vi "ParseXMLComment4Params.vi"(8 "error in":errorcluster, 11 "XML Comment":string) -> (0 "error out":errorcluster, 3 "ARINC Parameter":T1)   [LabVIEW 2011, in "AIT 429 Custom Device.lvlib"]
uses:
  AIT 429 Custom Device.lvlib
  Controls/ARINCParam.ctl
  <vilib>/xml/Close Reference(Node).vi
  Program Files (x86)/National Instruments/LabVIEW 2011/resource/objmgr/DOMUserDefRef.rc
  <vilib>/xml/NI_XML.lvlib
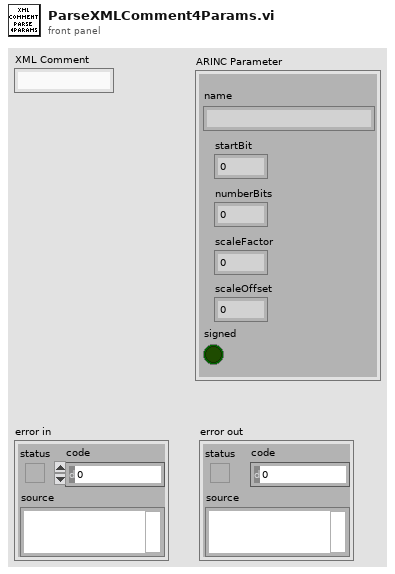
[diagram p1: front panel]
types:
  T1 = typedef "AIT 429 Custom Device.lvlib/ARINCParam.ctl" = cluster{"name":string, "startBit":i32, "numberBits":i32, "scaleFactor":dbl, "scaleOffset":dbl, "signed":bool}
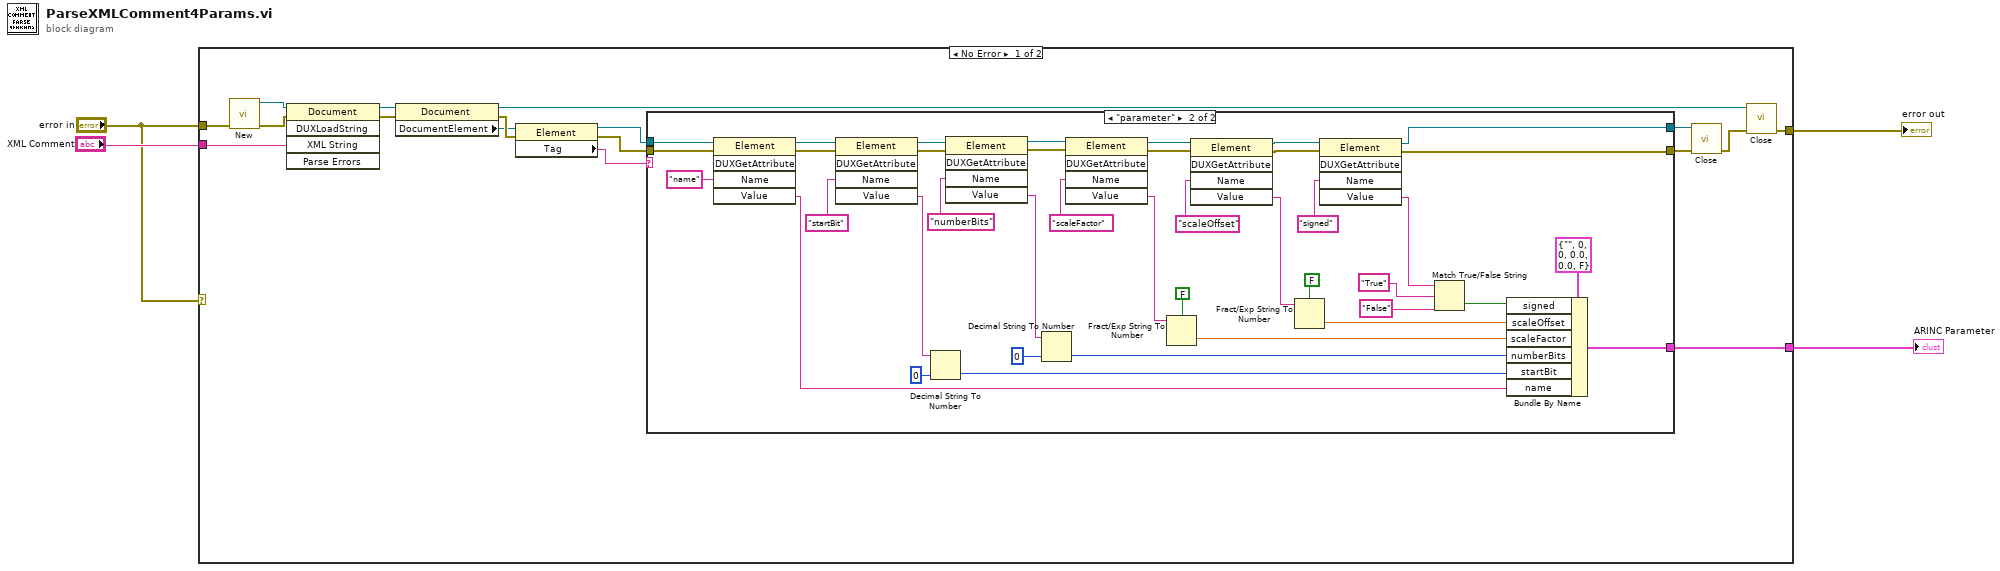
[diagram p0: block diagram]
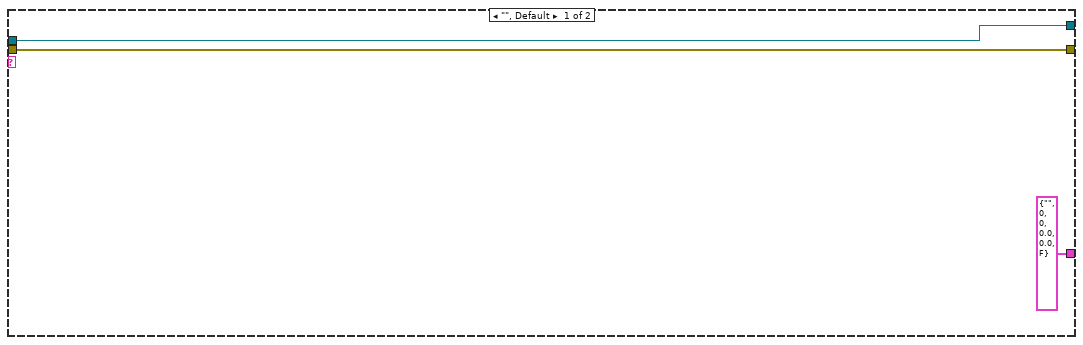
[diagram p2: hidden frame]
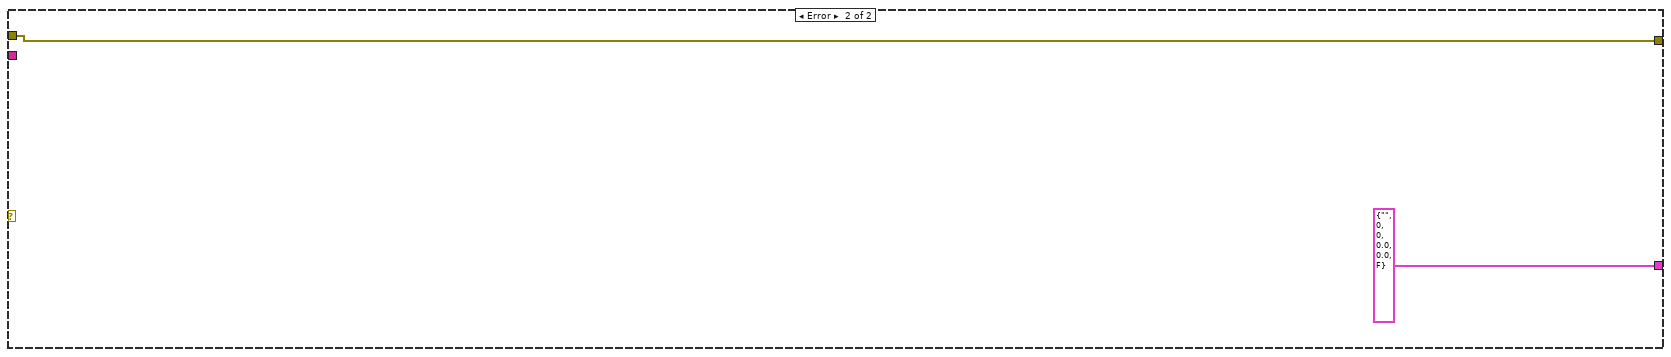
[diagram p3: hidden frame]
diagram:
  n1 = case shown="No Error" "error in" {
    tunnel: [w16 w65] -> w4
    tunnel: "XML Comment" -> [w9 _]
    tunnel: "error in" -> [w8 w65]
    tunnel: [w5 T1 {"name"="", "startBit"=0, "numberBits"=0, "scaleFactor"=0.0, "scaleOffset"=0.0, "signed"=FALSE} ("ARINC Parameter")] -> w2
    frame No Error {
      n2 = call <vilib>:"New.vi"("error in (no error)"=w8) -> ("error out"=w10:errorcluster, "DOM document out"=w7:refnum<k20>)  [unwired: 7 in]
      n3 = invoke class="Document" method="DUXLoadString"(reference=w7, error in=w10, "XML String"=w9) -> (reference out=w6:refnum<k20>, error out=w11:errorcluster)  [unwired: 2 in, 3 out]
      n4 = property on="Property Node" class="Document"(reference=w6, error in=w11) -> (reference out=w12:refnum<k20>, error out=w19:errorcluster, "DocumentElement"=w17:refnum<k20>)
      n5 = property class="Element"(reference=w17, error in=w19) -> (reference out=w18:refnum<k20>, error out=w20:errorcluster, "Tag"=w21:string)
      n6 = case shown="\"parameter\"" w21 {
        tunnel: [w23 w31] -> w14
        tunnel: [w24 w32] -> w15
        tunnel: w18 -> [w23 w62]
        tunnel: w20 -> [w24 w61]
        tunnel: [T1 {"name"="", "startBit"=0, "numberBits"=0, "scaleFactor"=0.0, "scaleOffset"=0.0, "signed"=FALSE} ("ARINC Parameter") w27] -> w5
        frame "", Default {
        }
        frame "parameter" {
          n7 = invoke on="Invoke Node" class="Element" method="DUXGetAttribute"(reference=w62, error in=w61, "Name"="name") -> (reference out=w60:refnum<k20>, error out=w59:errorcluster, "Value"=w57:string)  [unwired: 2 in, 2 out]
          n8 = invoke on="Invoke Node" class="Element" method="DUXGetAttribute"(reference=w60, error in=w59, "Name"="startBit") -> (reference out=w55:refnum<k20>, error out=w54:errorcluster, "Value"=w53:string)  [unwired: 2 in, 2 out]
          n9 = Decimal String To Number(string=w53, default (0L)=u32 0 ("default (0 I32)")) -> (number=w52:u32)  [unwired: 1 in, 1 out]
          n10 = invoke on="Invoke Node" class="Element" method="DUXGetAttribute"(reference=w55, error in=w54, "Name"="numberBits") -> (reference out=w48:refnum<k20>, error out=w47:errorcluster, "Value"=w50:string)  [unwired: 2 in, 2 out]
          n11 = Decimal String To Number(string=w50, default (0L)=u32 0 ("default (0 I32)")) -> (number=w49:u32)  [unwired: 1 in, 1 out]
          n12 = invoke on="Invoke Node" class="Element" method="DUXGetAttribute"(reference=w48, error in=w47, "Name"="scaleFactor") -> (reference out=w45:refnum<k20>, error out=w44:errorcluster, "Value"=w43:string)  [unwired: 2 in, 2 out]
          n13 = Fract/Exp String To Number(use system decimal point (T)=FALSE, string=w43) -> (number=w42:dbl)  [unwired: 2 in, 1 out]
          n14 = invoke on="Invoke Node" class="Element" method="DUXGetAttribute"(reference=w45, error in=w44, "Name"="scaleOffset") -> (reference out=w39:refnum<k20>, error out=w38:errorcluster, "Value"=w41:string)  [unwired: 2 in, 2 out]
          n15 = Fract/Exp String To Number(use system decimal point (T)=FALSE, string=w41) -> (number=w40:dbl)  [unwired: 2 in, 1 out]
          n16 = invoke on="Invoke Node" class="Element" method="DUXGetAttribute"(reference=w39, error in=w38, "Name"="signed") -> (reference out=w31:refnum<k20>, error out=w32:errorcluster, "Value"=w36:string)  [unwired: 2 in, 2 out]
          n17 = Match True/False String(2:"False" ("true string"), 3:"True" ("true string"), 4:w36) -> (0:w33:bool)  [unwired: 1 out]
          n18 = Bundle By Name(cluster=T1 {"name"="", "startBit"=0, "numberBits"=0, "scaleFactor"=0.0, "scaleOffset"=0.0, "signed"=FALSE} ("ARINC Parameter"), "signed"=w33, "scaleOffset"=w40, "scaleFactor"=w42, "numberBits"=w49, "startBit"=w52, "name"=w57) -> (w27:T1)
        }
      }
      n19 = call-poly <vilib>:"Close.vi"("error in (no error)"=w15, "node"=w14) -> ("error out"=w13:errorcluster)  [unwired: 7 out]
      n20 = call-poly <vilib>:"Close.vi"("error in (no error)"=w13, "node"=w12) -> ("error out"=w16:errorcluster)  [unwired: 7 out]
    }
    frame Error {
    }
  }
  "error out" <- w4
  "ARINC Parameter" <- w2
